vi "Create Handle Messages Method.vi"(8 "error in (no error)":errorcluster, 11 "Process Generator in":refnum<class "Process Generator.lvclass">) -> (0 "error out":errorcluster, 3 "Process Generator out":refnum<class "Process Generator.lvclass">)   [LabVIEW 2020, in "Process Generation.lvlib" / "Process Generator.lvclass"]
uses:
  Process Generator.lvclass
  <vilib>/Utility/traverseref.llb/TRef TravTarget.ctl
  Process Generator.lvclass/Process Generator.ctl
  <vilib>/Utility/traverseref.llb/VI Scripting - Traverse.lvlib
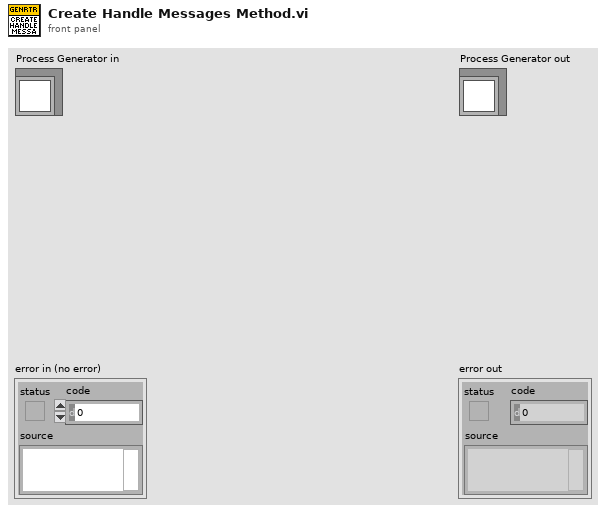
[diagram p1: front panel]
types:
  T1 = typedef "TRef TravTarget.ctl" = enum16{"FP", "BD", "Other"}
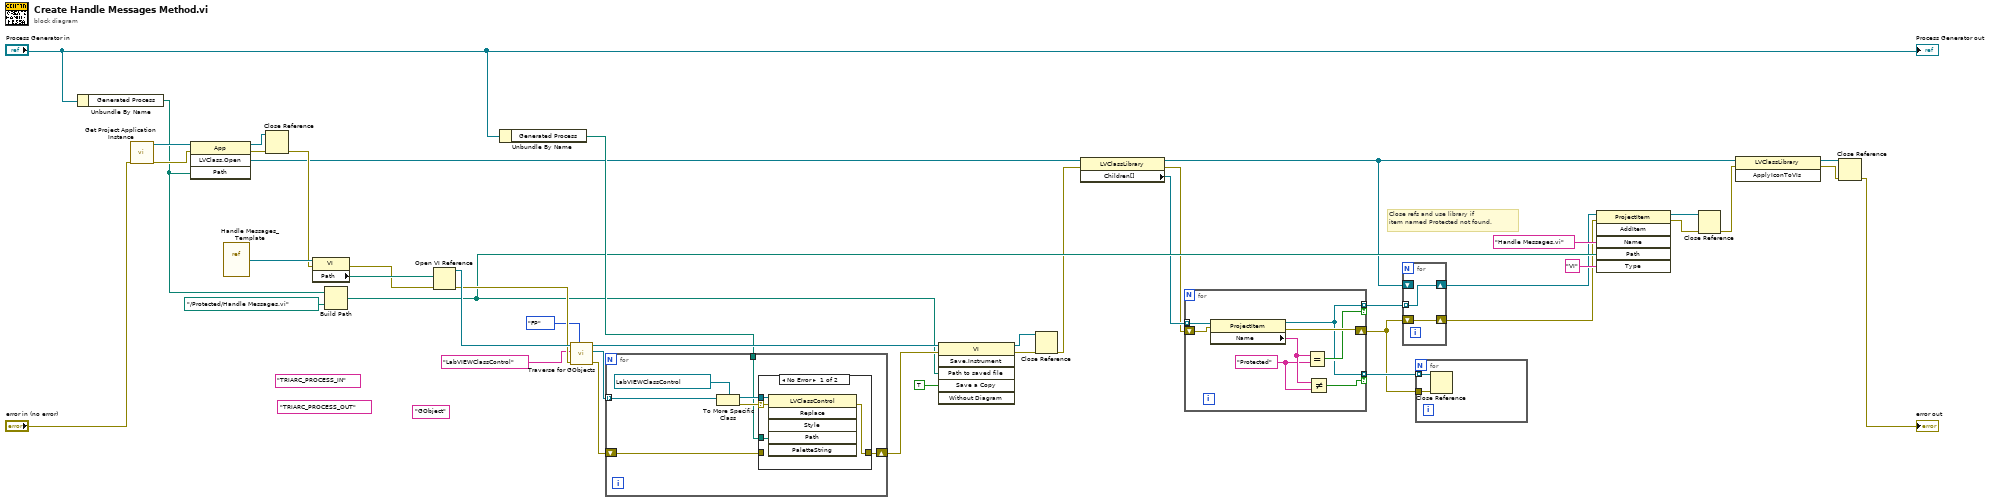
[diagram p0: block diagram]
diagram:
  (unwired) "GObject"
  (unwired) "TRIARC_PROCESS_OUT"
  (unwired) "TRIARC_PROCESS_IN"
  # "Close refs and use library if \nitem named Protected not found."
  n1 = Unbundle By Name("Process Generator in") -> ("Generated Process"=w40:path)
  n2 = call "Get Project Application Instance.vi"("error in (no error)"="error in (no error)") -> ("error out"=w42:errorcluster, "Application out"=w43:refnum<vi>)  [unwired: 9 in]
  n3 = invoke class="App" method="LVClass.Open"(reference=w43, error in=w42, "Path"=w40) -> (reference out=w16:refnum<vi>, error out=w32:errorcluster, "LVClass.Open"=w14:refnum<vi>)  [unwired: 1 in, 1 out]
  n4 = vi-ref "Handle Messages_Template.vi"() -> (w41:refnum<vi>)
  n5 = Close Reference(reference=w16, error in (no error)=w32) -> (error out=w17:errorcluster)
  n6 = property class="VI"(reference=w41, error in=w17) -> (error out=w31:errorcluster, "Path"=w34:path)  [unwired: 1 out]
  n7 = Build Path(base path=w40, name or relative path=path "../Protected/Handle Messages.vi") -> (appended path=w18:path)
  n8 = Open VI Reference(vi path=w34, error in (no error)=w31) -> (vi reference=w35:refnum<vi>, error out=w30:errorcluster)  [unwired: 4 in]
  n9 = Unbundle By Name("Process Generator in") -> ("Generated Process"=w20:path)
  n10 = call <vilib>:"Traverse for GObjects.vi"("Traverse Target"=TRef_TravTarget."FP", "error in (no error)"=w30, "Class Name"="LabVIEWClassControl", "VI Refnum"=w35) -> ("error out"=w22:errorcluster, "References"=w24:refnum<vi>[], "dup VI Refnum"=w26:refnum<vi>)  [unwired: 4 in, 1 out]
  n11 = for {
    tunnel: w24 -> [w50] mode=indexing
    tunnel: w20 -> [w46]
    shift-right: [w45] -> w23
    shift-left: w22 -> [w44]
    n12 = To More Specific Class(target class=refnum<vi> refnum ("reference out"), reference=w50) -> (specific class reference=w47:refnum<vi>, error out=w48:errorcluster)  [unwired: 1 in]
    n13 = case shown="No Error" w48 {
      selector: w48 -> [w54 _]
      tunnel: w47 -> [w53 _]
      tunnel: w46 -> [w52 _]
      tunnel: [w51 w55] -> w45
      tunnel: w44 -> [_ w55]
      frame No Error {
        n14 = invoke on="Invoke Node" class="LVClassControl" method="Replace"(reference=w53, error in=w54, "Path"=w52) -> (error out=w51:errorcluster)  [unwired: 3 in, 5 out]
      }
      frame Error {
      }
    }
  }
  n15 = invoke on="Invoke Node" class="VI" method="Save.Instrument"(reference=w26, error in=w23, "Path to saved file"=w18, "Save a Copy"=TRUE) -> (reference out=w27:refnum<vi>, error out=w28:errorcluster)  [unwired: 2 in, 4 out]
  n16 = Close Reference(reference=w27, error in (no error)=w28) -> (error out=w11:errorcluster)
  n17 = property class="LVClassLibrary"(reference=w14, error in=w11) -> (reference out=w5:refnum<vi>, error out=w12:errorcluster, "Children[]"=w13:refnum<vi>[])
  n18 = for {
    tunnel: w13 -> [w63] mode=indexing
    tunnel: [w59] -> w9 mode=indexing if=w60
    shift-right: [w62] -> w8
    shift-left: w12 -> [w61]
    tunnel: [w59] -> w10 mode=indexing if=w56
    w57 = "Protected"
    n19 = property class="ProjectItem"(reference=w63, error in=w61) -> (reference out=w59:refnum<vi>, error out=w62:errorcluster, "Name"=w58:string)
    n20 = Equal?(x=w58, y=w57) -> (x = y?=w60:bool)
    n21 = Not Equal?(x=w58, y=w57) -> (x != y?=w56:bool)
  }
  n22 = for {
    tunnel: w9 -> [w65] mode=indexing
    shift-right: [w65] -> w6
    shift-left: w5 -> [_]
    shift-right: [w64] -> w7
    shift-left: w8 -> [w64]
  }
  n23 = for {
    tunnel: w10 -> [w67] mode=indexing
    tunnel: w8 -> [w66]
    n24 = Close Reference(reference=w67, error in (no error)=w66) -> ()  [unwired: 1 out]
  }
  n25 = invoke class="ProjectItem" method="AddItem"(reference=w6, error in=w7, "Name"="Handle Messages.vi", "Path"=w18, "Type"="VI") -> (reference out=w37:refnum<vi>, error out=w38:errorcluster)  [unwired: 1 in, 4 out]
  n26 = Close Reference(reference=w37, error in (no error)=w38) -> (error out=w2:errorcluster)
  n27 = invoke class="LVClassLibrary" method="ApplyIconToVIs"(reference=w5, error in=w2) -> (reference out=w4:refnum<vi>, error out=w3:errorcluster)  [unwired: 1 in, 1 out]
  n28 = Close Reference(reference=w4, error in (no error)=w3) -> (error out=→"error out":errorcluster)
  "Process Generator out" <- "Process Generator in"
